vi "PH_gentec_Powermeter.set i Attr.vi"(0 "i ref in":refnum<vi>, 5 "error in":errorcluster) -> (14 "i ref out":refnum<vi>, 16 "i Attributes":T1 {"Current Sets"."Data Sampling Settings"."Time Stamp" items=["Off", "On"]; "Current Sets"."Data Sampling Settings"."Total Duration Unit" items=["Period", "Seconds", "Minutes", "Hours", "Days", "Weeks", "Continuous", "# of Points"]; "Current Sets"."Data Sampling Settings"."Total Duration" max=300 step=1; "Current Sets"."Data Sampling Settings"."Sample Period Unit" items=["Seconds", "Minutes", "Hours", "Days", "Weeks", "Pulses"]; "Current Sets"."Data Sampling Settings"."Sample Rate Unit" items=["per Second", "per Minute", "per Hour", "per Day", "% pulses"]; "Current Sets"."Data Sampling Settings"."Sample Rate" max=300 step=1; "Wanted Sets"."Data Sampling Settings"."Time Stamp" items=["Off", "On"]; "Wanted Sets"."Data Sampling Settings"."Total Duration Unit" items=["Period", "Seconds", "Minutes", "Hours", "Days", "Weeks", "Continuous", "# of Points"]; "Wanted Sets"."Data Sampling Settings"."Total Duration" max=300 step=1; "Wanted Sets"."Data Sampling Settings"."Sample Period Unit" items=["Seconds", "Minutes", "Hours", "Days", "Weeks", "Pulses"]; "Wanted Sets"."Data Sampling Settings"."Sample Rate Unit" items=["per Second", "per Minute", "per Hour", "per Day", "% pulses"]; "Wanted Sets"."Data Sampling Settings"."Sample Rate" max=300 step=1}, 19 "error out":errorcluster)   [LabVIEW 2014, in "PH_gentec_Powermeter.lvlib"]
doc: "This VI reads the DB entries and sets several attributes and GUI element settings."
uses:
  PH_gentec_Powermeter.lvlib
  PH_gentec_Powermeter.i attribute.ctl
  instr.lib/gentec-SOLO-PE/Driver/Type Defs/gentec-SOLO-PE.Statistics Data.ctl
  instr.lib/gentec-SOLO-PE/Driver/Type Defs/gentec-SOLO-PE.Configuration Values.ctl
  instr.lib/gentec-SOLO-PE/Driver/Type Defs/gentec-SOLO-PE.Scale.ctl
  instr.lib/gentec-SOLO-PE/Driver/Type Defs/gentec-SOLO-PE.Data Sampling Settings.ctl
  PH_gentec_Powermeter.Sets.ctl
  instr.lib/gentec-SOLO-PE/gentec-SOLO-PE - Driver.lvlib
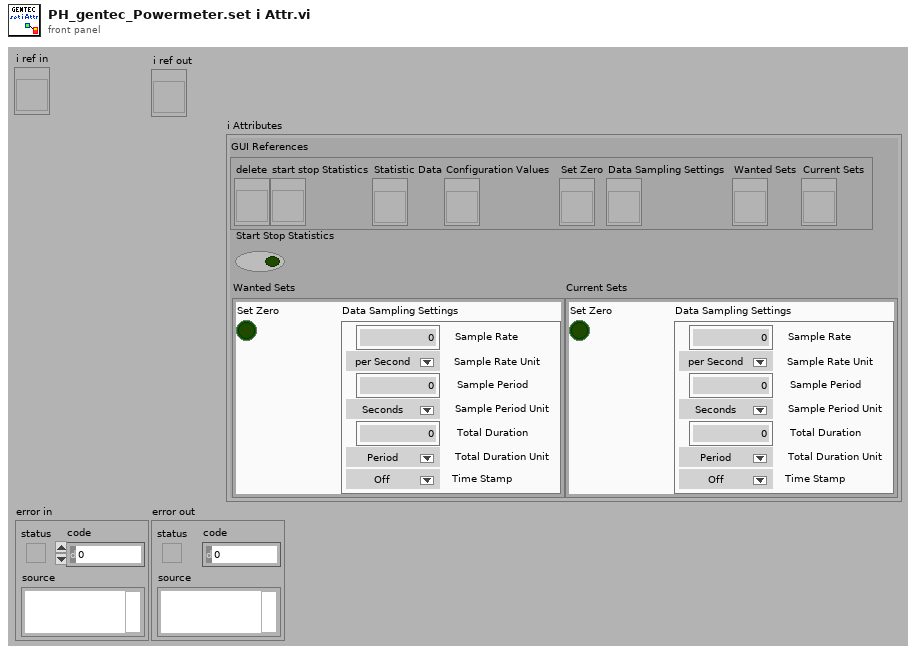
[diagram p1: front panel]
types:
  T1 = typedef "PH_gentec_Powermeter.lvlib/PH_gentec_Powermeter.i attribute.ctl" = cluster{"GUI References":cluster{"delete":refnum<vi>, "start stop Statistics":refnum<vi>, "Statistic Data":refnum<vi>, "Configuration Values":refnum<vi>, "Set Zero":refnum<vi>, "Data Sampling Settings":refnum<vi>, "Wanted Sets":refnum<vi>, "Current Sets":refnum<vi>}, "Start Stop Statistics":bool, "Wanted Sets":T2, "Current Sets":T2}
  T2 = typedef "PH_gentec_Powermeter.lvlib/PH_gentec_Powermeter.Sets.ctl" = cluster{"Data Sampling Settings":T3, "Set Zero":bool}
  T3 = typedef "gentec-SOLO-PE - Driver.lvlib/gentec-SOLO-PE.Data Sampling Settings.ctl" = cluster{"Sample Rate":u32, "Sample Rate Unit":u32, "Sample Period":u32, "Sample Period Unit":u32, "Total Duration":u32, "Total Duration Unit":u32, "Time Stamp":u32}
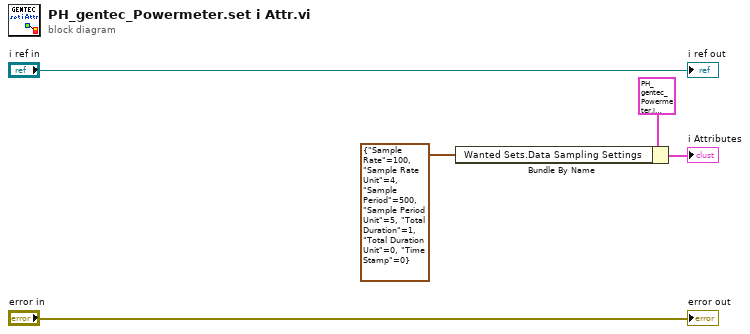
[diagram p0: block diagram]
diagram:
  n1 = Bundle By Name(cluster=T1 {"GUI References"={"delete"=refnum, "start stop Statistics"=refnum, "Statistic Data"=refnum, "Configuration Values"=refnum, "Set Zero"=refnum, "Data Sampling Settings"=refnum, "Wanted Sets"=refnum, "Current Sets"=refnum}, "Start Stop Statistics"=FALSE, "Wanted Sets"={"Data Sampling Settings"={"Sample Rate"=0, "Sample Rate Unit"=0, "Sample Period"=0, "Sample Period Unit"=0, "Total Duration"=0, "Total Duration Unit"=0, "Time Stamp"=0}, "Set Zero"=FALSE}, "Current Sets"={"Data Sampling Settings"={"Sample Rate"=0, "Sample Rate Unit"=0, "Sample Period"=0, "Sample Period Unit"=0, "Total Duration"=0, "Total Duration Unit"=0, "Time Stamp"=0}, "Set Zero"=FALSE}} ("i attribute"), "Wanted Sets.Data Sampling Settings"=T3 {"Sample Rate"=100, "Sample Rate Unit"=4, "Sample Period"=500, "Sample Period Unit"=5, "Total Duration"=1, "Total Duration Unit"=0, "Time Stamp"=0} ("Data Samling Settings")) -> (→"i Attributes":T1)
  "i ref out" <- "i ref in"
  "error out" <- "error in"
